vi "test-numerical-jacobian-CxDu-func.vi"(8 "U":T1, 9 "D":T1, 10 "X":T1, 11 "C":T1) -> (0 "Error":bool, 3 "OUT":T1)   [LabVIEW 2019]
uses:
  <vilib>/Analysis/Matrix/Datatypes/RealMatrix.ctl
  <vilib>/Analysis/baseanly.llb/Real A x B.vi
  <vilib>/Analysis/Matrix/Numeric/Add/Add - RM,RM.vi
  <vilib>/Analysis/NI_AALBase.lvlib
  <vilib>/Analysis/Matrix/NI_Matrix.lvlib
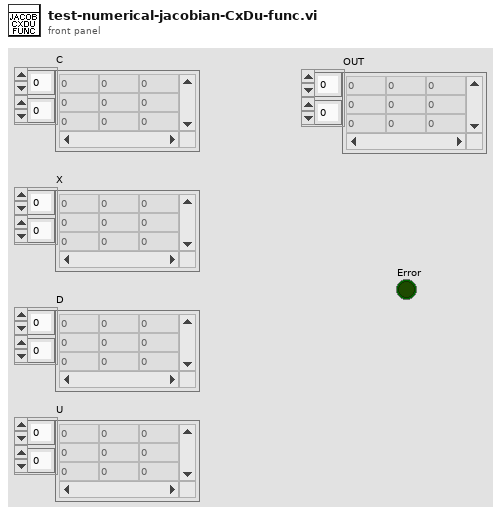
[diagram p1: front panel]
types:
  T1 = typedef "NI_Matrix.lvlib/RealMatrix.ctl" = dbl[][]
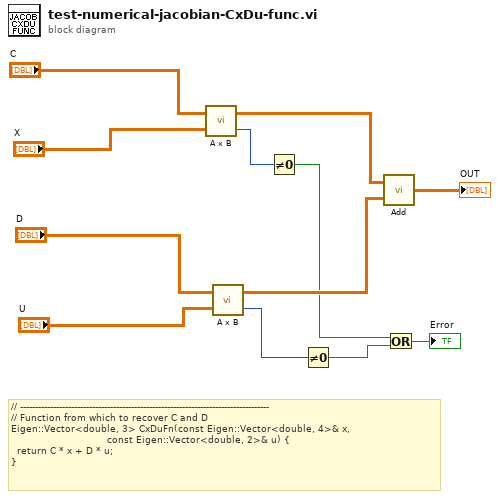
[diagram p0: block diagram]
diagram:
  # "// -----------------------------------------------------------------------------------\n// Function from which to recover C and D\nEigen::Vector<double, 3> CxDuFn(const Eigen::Vector<double, 4>& x,\n                                const Eigen::Vector<double, 2>& u) {\n  return C * x + D * u;\n}"
  n1 = call-poly <vilib>:"A x B.vi"("B"="X", "A"="C") -> ("error"=w7:i32, "A x B"=w8:T1)
  n2 = call-poly <vilib>:"A x B.vi"("B"="U", "A"="D") -> ("error"=w6:i32, "A x B"=w5:T1)
  n3 = Not Equal To 0?(x=w7) -> (x != 0?=w2:bool)
  n4 = Not Equal To 0?(x=w6) -> (x != 0?=w3:bool)
  n5 = call-poly <vilib>:"Add.vi"("Real Matrix B"=w5, "Real Matrix A"=w8) -> ("A + B"=→"OUT":T1)
  n6 = Or(x=w2, y=w3) -> (x .or. y?=→"Error":bool)
